vi "WaveformComponent, Add Uniform White Noise.vi"(0 "waveform":waveform(dbl)={"t0"=timestamp(3474820848.0780005 s since 1904-01-01), "dt"=nan, "Y"=[]}, 1 "level (1.0)":dbl[unit]=0.5 format="%.3f") -> (3 "waveform out":waveform(dbl)={"t0"=timestamp(-9593225999.921999 s since 1904-01-01), "dt"=nan, "Y"=[]})   [LabVIEW 2010]
uses:
  <vilib>/Analysis/NI_AALBase.lvlib
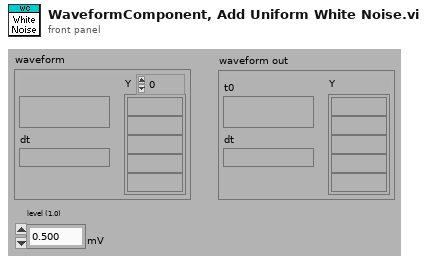
[diagram p1: front panel]
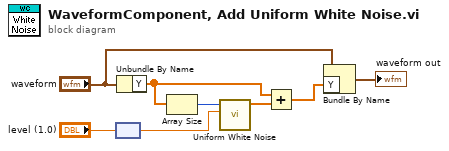
[diagram p0: block diagram]
diagram:
  n1 = node("level (1.0)") -> (w1:dbl)
  n2 = Unbundle By Name("waveform") -> ("Y"=w3:dbl[])
  n3 = Array Size(array=w3) -> (size(s)=w6:i32)
  n4 = call <vilib>:"Uniform White Noise.vi"("amplitude"=w1, "samples"=w6) -> ("uniform white noise"=w4:dbl[])  [unwired: 8 in, 1 out]
  n5 = Add(x=w3, y=w4) -> (x+y=w2:dbl[])
  n6 = Bundle By Name(cluster="waveform", "Y"=w2) -> (→"waveform out":waveform(dbl))
